vi "enqueue.vi"(6 "priority (f)":bool, 8 "error in (no error)":errorcluster, 10 "states":T1, 11 "EventDaemon in":refnum<class "MemoryManager.lvclass">) -> (0 "error out":errorcluster, 3 "EventDaemon out":refnum<class "MemoryManager.lvclass">)   [LabVIEW 2024, in "MemoryManager.lvclass"]
doc: "Enqueues private states for daemon. Set priority to True to enqueue to the front."
uses:
  MemoryManager.lvclass
  states--enum.ctl
  MemoryManager.lvclass/MemoryManager.ctl
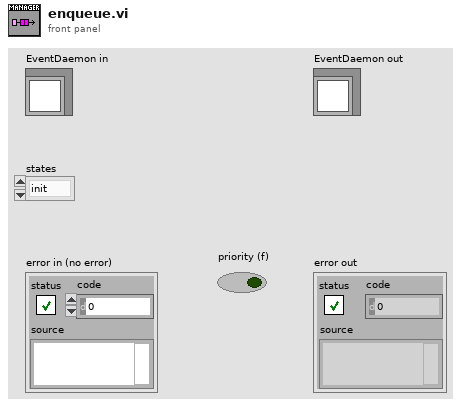
[diagram p1: front panel]
types:
  T1 = typedef "MemoryManager.lvclass/states--enum.ctl" = enum16{"init", "default", "error handler", "exit"}
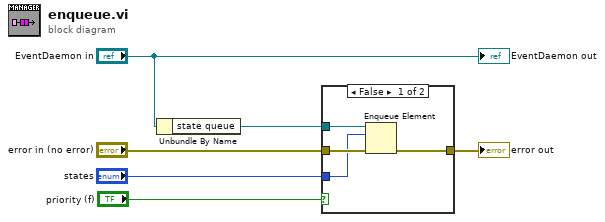
[diagram p0: block diagram]
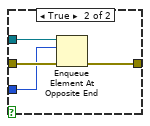
[diagram p2: hidden frame]
diagram:
  n1 = Unbundle By Name("EventDaemon in") -> ("state queue"=w5:refnum<queue>)
  n2 = case shown="False" "priority (f)" {
    tunnel: w5 -> [w10 w14]
    tunnel: "error in (no error)" -> [w9 w13]
    tunnel: [w8 w12] -> w3
    tunnel: "states" -> [w7 w11]
    frame False {
      n3 = Enqueue Element(queue=w10, element=w7, error in (no error)=w9) -> (error out=w8:errorcluster)  [unwired: 1 in, 2 out]
    }
    frame True {
      n4 = Enqueue Element At Opposite End(queue=w14, element=w11, error in (no error)=w13) -> (error out=w12:errorcluster)  [unwired: 1 in, 2 out]
    }
  }
  "error out" <- w3
  "EventDaemon out" <- "EventDaemon in"
